vi "setUp.vi"(8 "error in (no error)":errorcluster, 11 "TestObservableData In":refnum<class "TestObservableData.lvclass">) -> (0 "error out":errorcluster, 3 "TestObservableData Out":refnum<class "TestObservableData.lvclass">)   [LabVIEW 2015, in "TestObservableData.lvclass"]
doc: "setUp runs prior to the test method during test execution. Use this method to initialize any object data required by your tests."
uses:
  TestObservableData.lvclass
  LeakyViewModel/LeakyViewModel.lvclass
  Framework/IViewable/IViewable/IViewable.lvclass
  MockModel/MockModel/MockModelOneShotPublish/MockModelOneShotPublish.lvclass
  Framework/Mediator/Mediator/Mediator.lvclass
  Framework/IViewModel/IViewModel/IViewModel.lvclass/IViewModel.ctl
  Framework/IViewManager/IViewManager Messages/Launch Nested Views Msg/Launch Nested Views Msg.lvclass/Launch Nested Views Msg.ctl
  Framework/IViewManager/IViewManager/IViewManager.lvclass/IViewManager.ctl
  TestObservableData.lvclass/TestObservableData.ctl
  LeakyViewModel Messages/GiveMeYourMediatorQueue Msg/GiveMeYourMediatorQueue Msg.lvclass/GiveMeYourMediatorQueue Msg.ctl
  <vilib>/ActorFramework/Message Enqueuer/Message Enqueuer.lvclass/Message Enqueuer.ctl
  Framework/IViewManager/IViewManager Messages/Launch Nested Views Msg/Build Launch Nested Views Msg.vi
  Framework/IViewManager/IViewManager/Write Startup Launch Nested Views Msg.vi
  <vilib>/ActorFramework/Message Enqueuer/Enqueue.vi
  <vilib>/ActorFramework/Message Priority Queue/Priority Enqueue.vi
  Framework/IViewManager/IViewManager Messages/Launch Nested Views Msg/Launch Nested Views Msg.lvclass
  LeakyViewModel Messages/GiveMeYourMediatorQueue Msg/GiveMeYourMediatorQueue Msg.lvclass
  <vilib>/addons/_JKI Toolkits/VI Tester/TestCase.llb/TestCase.lvclass
  Framework/IViewModel/IViewModel/IViewModel.lvclass
  <vilib>/ActorFramework/Actor/Actor.lvclass
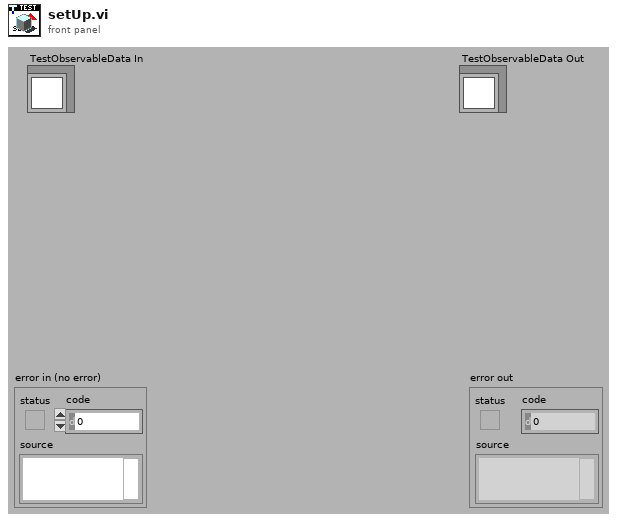
[diagram p1: front panel]
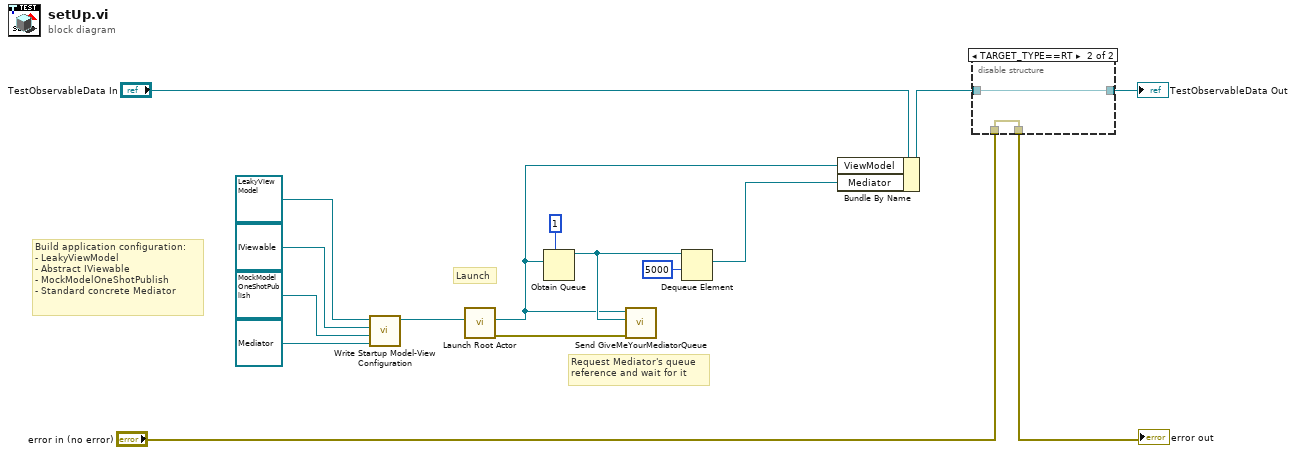
[diagram p0: block diagram]
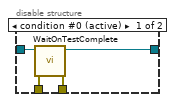
[diagram p2: hidden frame]
diagram:
  # "Request Mediator's queue\nreference and wait for it"
  # "Launch"
  # "Build application configuration:\n- LeakyViewModel\n- Abstract IViewable\n- MockModelOneShotPublish\n- Standard concrete Mediator"
  n1 = call "Write Startup Model-View Configuration.vi"("Mediator"=refnum<class "Mediator.lvclass"> refnum, "Model"=refnum<class "MockModelOneShotPublish.lvclass"> refnum, "Startup View Configuration"=refnum<class "IViewable.lvclass"> refnum, "IViewModel In"=refnum<class "LeakyViewModel.lvclass"> refnum) -> ("IViewModel Out"=w7:refnum<class "LeakyViewModel.lvclass">)  [unwired: 7 in]
  n2 = call <vilib>:"Launch Root Actor.vi"("Actor"=w7) -> ("error out"=w5:errorcluster, "Actor's Enqueuer"=w2:refnum<class "Message Enqueuer.lvclass">)  [unwired: 9 in]
  n3 = Obtain Queue(max queue size (-1, unlimited)=1, element data type=w2) -> (queue out=w4:refnum<queue>)  [unwired: 3 in, 2 out]
  n4 = call "Send GiveMeYourMediatorQueue.vi"("error in (no error)"=w5, "Reply Queue"=w4, "Message Enqueuer"=w2) -> ()  [unwired: 7 in, 2 out]
  n5 = Dequeue Element(queue=w4, timeout in ms (-1)=5000) -> (element=w1:refnum<class "Message Enqueuer.lvclass">)  [unwired: 1 in, 3 out]
  n6 = Bundle By Name(cluster="TestObservableData In", "ViewModel"=w2, "Mediator"=w1) -> (w12:refnum<class "TestObservableData.lvclass">)
  n7 = disable-structure shown="TARGET_TYPE==RT" {
    disable-tunnel: "error in (no error)" -> [w20 w21]
    disable-tunnel: [w19 w21] -> w15
    disable-tunnel: [w18 w22] -> w13
    disable-tunnel: w12 -> [w17 w22]
    frame condition #0 (active) {
      n8 = call <vilib>:"WaitOnTestComplete.vi"("error in (no error)"=w20, "TestCase in"=w17) -> ("error out"=w19:errorcluster, "TestCase out"=w18:refnum<class "TestObservableData.lvclass">)  [unwired: 8 in]
    }
    frame condition #1 {
    }
  }
  "error out" <- w15
  "TestObservableData Out" <- w13
